vi "Master Property Node.vi"   [LabVIEW 2017]
doc: "Sets or writes properties for a Modbus master instance. Use this node to set the read operation timeout, write operation timeout, or both timeouts on a Modbus slave and to set the identification of a Modbus slave."
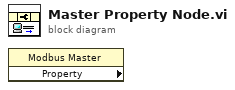
[diagram p0: block diagram]
diagram:
  n1 = property class="Modbus Master" props=[]() -> ()  [unwired: 2 in, 3 out]
